vi "calcWaypoints.vi"(3 "boat x":dbl, 4 "Clearance":dbl, 5 "Mission Type":T1) -> (0 "y 3":dbl, 1 "x 2":dbl, 2 "y 1":dbl)   [LabVIEW 2013]
doc: "Given wind from +x and the bouy at (0,0), calculate the reletive locations of the three waypoints.\n\nKaitlin Gallagher and Rocco DeVerdi\n(2/8/2015)"
uses:
  Data/TypeDefs/MissionTypeControl.ctl
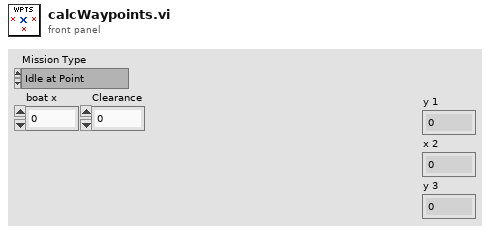
[diagram p1: front panel]
types:
  T1 = typedef "MissionTypeControl.ctl" = enum16{"Idle at Point", "Drive to Waypoint", "Round Buoy to Port", "Round Buoy to Starboard", "Pass Between Buoys", "Station Keeping"}
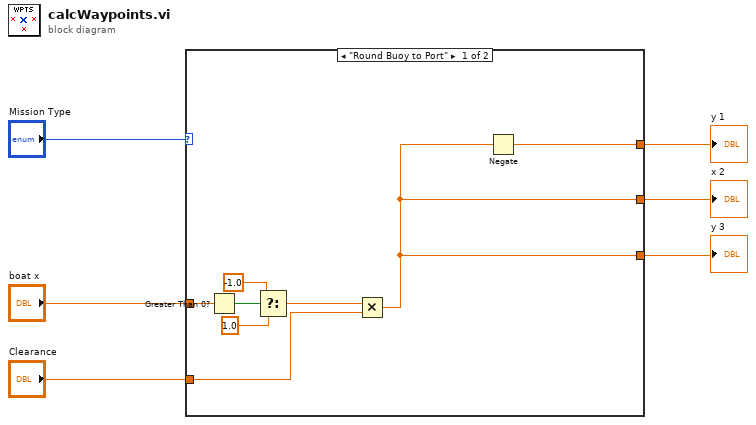
[diagram p0: block diagram]
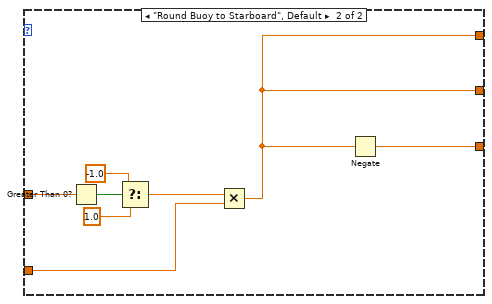
[diagram p2: hidden frame]
diagram:
  n1 = case shown="\"Round Buoy to Port\"" "Mission Type" {
    tunnel: "boat x" -> [w10 w21]
    tunnel: "Clearance" -> [w9 w17]
    tunnel: [w8 w16] -> w3
    tunnel: [w7 w16] -> w2
    tunnel: [w7 w15] -> w1
    frame "Round Buoy to Port" {
      n2 = Greater Than 0?(x=w10) -> (x > 0?=w11:bool)
      n3 = Select(t=-1.0, s=w11, f=1.0) -> (s? t:f=w14:dbl)
      n4 = Multiply(x=w14, y=w9) -> (x*y=w7:dbl)
      n5 = Negate(x=w7) -> (-x=w8:dbl)
    }
    frame "Round Buoy to Starboard", Default {
      n6 = Greater Than 0?(x=w21) -> (x > 0?=w22:bool)
      n7 = Select(t=-1.0, s=w22, f=1.0) -> (s? t:f=w18:dbl)
      n8 = Multiply(x=w18, y=w17) -> (x*y=w16:dbl)
      n9 = Negate(x=w16) -> (-x=w15:dbl)
    }
  }
  "x 2" <- w2
  "y 1" <- w3
  "y 3" <- w1
